vi "相对标准偏差判断.vi"(9 "实测值":sgl, 10 "相对标准偏差":dbl, 11 "标样值":dbl) -> (3 "合格？":bool)   [LabVIEW 2016, in "斯坦道通用流路CODmn.lvlib"]
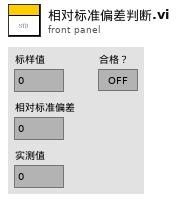
[diagram p1: front panel]
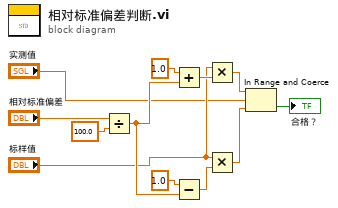
[diagram p0: block diagram]
diagram:
  n1 = Divide(x="相对标准偏差", y=100.0) -> (x/y=w9:dbl)
  n2 = Add(x=1.0, y=w9) -> (x+y=w7:dbl)
  n3 = Subtract(x=1.0, y=w9) -> (x-y=w6:dbl)
  n4 = Multiply(x="标样值", y=w7) -> (x*y=w4:dbl)
  n5 = Multiply(x="标样值", y=w6) -> (x*y=w3:dbl)
  n6 = In Range and Coerce(upper limit=w4, x="实测值", lower limit=w3) -> (In Range?=→"合格？":bool)  [unwired: 1 out]
